vi "Main_05A.vi"() -> ()   [LabVIEW 2024]
panel:
  out "Page Array":cluster{"Array":i32[]}[](array[cluster])
  out "Rules":i32[][](array[numeric])
  out "Answer 6267":u32
  in  "Puzzle":string="57|32\n67|77\n67|23\n54|27\n54|35\n54|99\n27|63\n27|83\n27|14\n27|47\n83|96\n83|25\n83|45\n83|33\n83|82\n46|81\n46|67\n46|27\n46|72\n46|21\n46|73\n85|54\n85|99\n85|98\n85|28\n85|53\n85|27\n85|63\n76|69\n76|21\n76|54\n76|48\n76|92\n76|81\n76|62\n76|23\n51|75\n51|68\n51|25\n51|72\n51|62\n51|96\n51|21\n51|11\n51|27\n24|77\n24|63\n24|76\n24|72\n24|51\n24|14\n24|39\n24|18\n24|62\n24|67\n77|53\n77|57\n77|75\n77|36\n77|11\n77|23\n77|69\n77|96\n77|85\n77|52\n77|81\n45|23\n45|73\n45|54\n45|81\n45|36\n45|27\n45|65\n45|96\n45|76\n45|33\n45|52\n45|46\n11|61\n11|19\n11|39\n11|94\n11|98\n11|54\n11|56\n11|92\n11|24\n11|27\n11|43\n11|69\n11|28\n18|43\n18|76\n18|47\n18|72\n18|39\n18|25\n18|63\n18|14\n18|62\n18|32\n18|67\n18|94\n18|96\n18|77\n33|77\n33|36\n33|54\n33|73\n33|96\n33|75\n33|28\n33|23\n33|11\n33|81\n33|68\n33|65\n33|46\n33|52\n33|85\n36|69\n36|65\n36|52\n36|75\n36|48\n36|76\n36|54\n36|19\n36|68\n36|81\n36|57\n36|73\n36|56\n36|62\n36|21\n36|92\n52|73\n52|48\n52|85\n52|83\n52|23\n52|27\n52|57\n52|11\n52|31\n52|92\n52|28\n52|19\n52|54\n52|75\n52|99\n52|65\n52|24\n63|33\n63|65\n63|32\n63|35\n63|52\n63|51\n63|62\n63|45\n63|72\n63|82\n63|46\n63|96\n63|77\n63|47\n63|67\n63|23\n63|36\n63|14\n73|27\n73|99\n73|21\n73|63\n73|92\n73|98\n73|83\n73|85\n73|69\n73|39\n73|54\n73|11\n73|53\n73|32\n73|61\n73|19\n73|18\n73|57\n73|48\n19|24\n19|47\n19|82\n19|32\n19|46\n19|39\n19|92\n19|14\n19|33\n19|69\n19|83\n19|94\n19|48\n19|18\n19|57\n19|61\n19|51\n19|99\n19|56\n19|63\n99|72\n99|13\n99|14\n99|96\n99|82\n99|76\n99|35\n99|18\n99|61\n99|46\n99|39\n99|36\n99|33\n99|77\n99|51\n99|67\n99|47\n99|43\n99|94\n99|63\n99|24\n47|72\n47|52\n47|75\n47|65\n47|14\n47|96\n47|46\n47|11\n47|33\n47|85\n47|73\n47|67\n47|51\n47|82\n47|81\n47|13\n47|25\n47|77\n47|76\n47|36\n47|23\n47|62\n35|72\n35|65\n35|81\n35|47\n35|36\n35|52\n35|75\n35|62\n35|45\n35|96\n35|33\n35|46\n35|67\n35|13\n35|77\n35|76\n35|85\n35|23\n35|73\n35|51\n35|25\n35|14\n35|68\n94|13\n94|47\n94|68\n94|65\n94|82\n94|51\n94|36\n94|43\n94|67\n94|76\n94|46\n94|96\n94|35\n94|45\n94|81\n94|33\n94|72\n94|62\n94|14\n94|23\n94|25\n94|77\n94|52\n94|73\n69|82\n69|83\n69|61\n69|43\n69|35\n69|46\n69|63\n69|25\n69|67\n69|14\n69|47\n69|33\n69|24\n69|32\n69|56\n69|39\n69|72\n69|51\n69|94\n69|92\n69|48\n69|99\n69|45\n69|18\n96|62\n96|75\n96|73\n96|85\n96|57\n96|65\n96|69\n96|31\n96|23\n96|76\n96|19\n96|36\n96|81\n96|11\n96|53\n96|28\n96|27\n96|56\n96|68\n96|52\n96|21\n96|48\n96|98\n96|54\n61|13\n61|52\n61|62\n61|67\n61|35\n61|51\n61|82\n61|39\n61|36\n61|77\n61|45\n61|63\n61|32\n61|76\n61|14\n61|72\n61|94\n61|47\n61|46\n61|43\n61|33\n61|18\n61|96\n61|25\n68|21\n68|98\n68|18\n68|83\n68|57\n68|28\n68|73\n68|53\n68|99\n68|19\n68|69\n68|63\n68|11\n68|92\n68|85\n68|27\n68|48\n68|39\n68|61\n68|75\n68|56\n68|54\n68|24\n68|31\n53|82\n53|47\n53|69\n53|24\n53|32\n53|61\n53|63\n53|31\n53|39\n53|14\n53|92\n53|18\n53|98\n53|56\n53|83\n53|19\n53|99\n53|33\n53|94\n53|57\n53|35\n53|48\n53|45\n53|43\n23|24\n23|21\n23|28\n23|65\n23|73\n23|48\n23|98\n23|75\n23|31\n23|92\n23|19\n23|69\n23|56\n23|68\n23|53\n23|85\n23|57\n23|99\n23|27\n23|83\n23|81\n23|61\n23|11\n23|54\n21|98\n21|92\n21|31\n21|48\n21|43\n21|57\n21|35\n21|69\n21|56\n21|82\n21|39\n21|63\n21|94\n21|61\n21|53\n21|47\n21|28\n21|19\n21|24\n21|27\n21|83\n21|18\n21|99\n21|32\n72|11\n72|53\n72|76\n72|52\n72|85\n72|68\n72|13\n72|19\n72|27\n72|54\n72|23\n72|57\n72|36\n72|31\n72|21\n72|28\n72|73\n72|77\n72|98\n72|96\n72|81\n72|75\n72|65\n72|62\n14|72\n14|73\n14|77\n14|76\n14|52\n14|25\n14|11\n14|96\n14|51\n14|65\n14|67\n14|62\n14|13\n14|36\n14|21\n14|75\n14|68\n14|33\n14|81\n14|23\n14|46\n14|85\n14|45\n14|54\n98|43\n98|56\n98|47\n98|61\n98|24\n98|39\n98|69\n98|63\n98|32\n98|57\n98|51\n98|33\n98|83\n98|18\n98|35\n98|82\n98|48\n98|94\n98|99\n98|92\n98|19\n98|46\n98|45\n98|14\n82|96\n82|81\n82|23\n82|14\n82|13\n82|76\n82|73\n82|68\n82|77\n82|75\n82|33\n82|65\n82|11\n82|72\n82|36\n82|46\n82|67\n82|52\n82|51\n82|25\n82|54\n82|85\n82|45\n82|62\n13|68\n13|81\n13|73\n13|65\n13|54\n13|57\n13|52\n13|28\n13|62\n13|76\n13|23\n13|75\n13|36\n13|53\n13|21\n13|56\n13|69\n13|98\n13|31\n13|96\n13|27\n13|85\n13|11\n13|19\n65|98\n65|24\n65|81\n65|73\n65|31\n65|48\n65|28\n65|11\n65|53\n65|99\n65|27\n65|19\n65|18\n65|92\n65|85\n65|21\n65|61\n65|54\n65|83\n65|69\n65|56\n65|75\n65|68\n65|57\n39|25\n39|96\n39|47\n39|65\n39|35\n39|33\n39|72\n39|36\n39|52\n39|77\n39|94\n39|45\n39|23\n39|13\n39|46\n39|76\n39|14\n39|82\n39|62\n39|32\n39|51\n39|67\n39|43\n39|63\n62|85\n62|28\n62|99\n62|23\n62|53\n62|19\n62|31\n62|81\n62|57\n62|54\n62|21\n62|48\n62|65\n62|83\n62|98\n62|75\n62|11\n62|52\n62|69\n62|56\n62|92\n62|27\n62|68\n62|73\n81|75\n81|28\n81|57\n81|56\n81|53\n81|48\n81|85\n81|11\n81|21\n81|92\n81|99\n81|68\n81|27\n81|24\n81|98\n81|61\n81|39\n81|31\n81|54\n81|83\n81|73\n81|18\n81|19\n81|69\n56|25\n56|35\n56|82\n56|32\n56|94\n56|67\n56|99\n56|33\n56|48\n56|18\n56|24\n56|47\n56|46\n56|39\n56|83\n56|72\n56|45\n56|61\n56|63\n56|77\n56|51\n56|43\n56|14\n56|92\n43|62\n43|72\n43|73\n43|51\n43|96\n43|35\n43|45\n43|33\n43|52\n43|67\n43|65\n43|46\n43|23\n43|68\n43|76\n43|14\n43|13\n43|82\n43|47\n43|81\n43|85\n43|25\n43|36\n43|77\n48|63\n48|33\n48|14\n48|32\n48|61\n48|18\n48|83\n48|43\n48|24\n48|45\n48|72\n48|13\n48|92\n48|51\n48|67\n48|47\n48|35\n48|99\n48|82\n48|94\n48|25\n48|77\n48|39\n48|46\n28|98\n28|14\n28|53\n28|56\n28|45\n28|24\n28|47\n28|69\n28|99\n28|82\n28|61\n28|39\n28|43\n28|18\n28|63\n28|31\n28|35\n28|32\n28|83\n28|92\n28|48\n28|94\n28|57\n28|19\n25|77\n25|28\n25|19\n25|75\n25|27\n25|76\n25|21\n25|31\n25|98\n25|23\n25|72\n25|54\n25|96\n25|85\n25|52\n25|81\n25|53\n25|62\n25|13\n25|68\n25|36\n25|11\n25|65\n25|73\n75|28\n75|53\n75|83\n75|69\n75|11\n75|99\n75|24\n75|31\n75|56\n75|21\n75|98\n75|54\n75|19\n75|32\n75|94\n75|61\n75|43\n75|18\n75|39\n75|48\n75|63\n75|92\n75|27\n75|57\n92|47\n92|25\n92|35\n92|83\n92|77\n92|67\n92|72\n92|51\n92|46\n92|24\n92|99\n92|32\n92|13\n92|82\n92|18\n92|63\n92|61\n92|33\n92|96\n92|94\n92|39\n92|43\n92|45\n92|14\n31|24\n31|35\n31|63\n31|83\n31|39\n31|57\n31|45\n31|94\n31|32\n31|43\n31|48\n31|18\n31|82\n31|56\n31|14\n31|98\n31|99\n31|69\n31|33\n31|47\n31|46\n31|92\n31|19\n31|61\n32|76\n32|65\n32|25\n32|33\n32|67\n32|68\n32|13\n32|82\n32|96\n32|47\n32|23\n32|52\n32|14\n32|72\n32|51\n32|94\n32|77\n32|43\n32|81\n32|46\n32|35\n32|36\n32|62\n32|45\n57|92\n57|45\n57|14\n57|63\n57|18\n57|33\n57|82\n57|47\n57|83\n57|99\n57|94\n57|35\n57|56\n57|25\n57|43\n57|69\n57|46\n57|61\n57|39\n57|51\n57|48\n57|24\n57|67\n67|25\n67|53\n67|65\n67|98\n67|27\n67|62\n67|13\n67|31\n67|75\n67|52\n67|72\n67|36\n67|11\n67|54\n67|73\n67|21\n67|81\n67|28\n67|76\n67|96\n67|85\n67|68\n54|56\n54|31\n54|69\n54|57\n54|98\n54|94\n54|61\n54|24\n54|92\n54|47\n54|53\n54|43\n54|19\n54|28\n54|18\n54|83\n54|32\n54|63\n54|21\n54|39\n54|48\n27|19\n27|24\n27|94\n27|35\n27|18\n27|56\n27|31\n27|99\n27|43\n27|82\n27|57\n27|39\n27|32\n27|98\n27|53\n27|28\n27|92\n27|48\n27|69\n27|61\n83|18\n83|67\n83|61\n83|13\n83|14\n83|94\n83|36\n83|72\n83|24\n83|39\n83|77\n83|35\n83|99\n83|43\n83|32\n83|51\n83|46\n83|63\n83|47\n46|25\n46|52\n46|36\n46|68\n46|13\n46|76\n46|96\n46|77\n46|11\n46|51\n46|75\n46|85\n46|28\n46|54\n46|23\n46|65\n46|62\n46|53\n85|94\n85|11\n85|21\n85|57\n85|69\n85|56\n85|24\n85|18\n85|31\n85|39\n85|92\n85|32\n85|83\n85|19\n85|48\n85|61\n85|75\n76|98\n76|52\n76|53\n76|85\n76|57\n76|68\n76|56\n76|28\n76|83\n76|19\n76|11\n76|65\n76|75\n76|31\n76|73\n76|27\n51|54\n51|36\n51|77\n51|52\n51|28\n51|23\n51|67\n51|13\n51|31\n51|76\n51|85\n51|81\n51|65\n51|53\n51|73\n24|94\n24|33\n24|25\n24|96\n24|32\n24|43\n24|35\n24|61\n24|13\n24|45\n24|82\n24|36\n24|46\n24|47\n77|31\n77|21\n77|76\n77|65\n77|98\n77|27\n77|54\n77|73\n77|28\n77|13\n77|19\n77|62\n77|68\n45|13\n45|51\n45|77\n45|68\n45|62\n45|72\n45|11\n45|75\n45|85\n45|67\n45|25\n45|21\n11|63\n11|21\n11|83\n11|35\n11|32\n11|53\n11|48\n11|57\n11|31\n11|99\n11|18\n18|35\n18|23\n18|33\n18|82\n18|51\n18|45\n18|13\n18|36\n18|52\n18|46\n33|13\n33|51\n33|21\n33|25\n33|72\n33|62\n33|67\n33|76\n33|27\n36|53\n36|27\n36|23\n36|98\n36|28\n36|85\n36|11\n36|31\n52|69\n52|53\n52|98\n52|21\n52|68\n52|81\n52|56\n63|13\n63|81\n63|43\n63|94\n63|76\n63|25\n73|28\n73|24\n73|75\n73|56\n73|31\n19|43\n19|67\n19|45\n19|35\n99|25\n99|45\n99|32\n47|68\n47|45\n35|82\n\n46,51,67,25,72,77,13,96,36,76,52,23,65,81,68,73,85,75,11,54,21,27,28\n68,73,85,75,11,54,21,28,31,19,57,69,56,48,92,83,99,24,61,18,39\n83,99,24,61,63,32,94,35,47,82,14,45,33,46,51,67,25,72,77,13,96\n19,81,75,36,27,96,11\n75,11,54,21,28,31,98,19,56,92,83,99,24,18,63,32,94\n62,23,85,75,27,31,19,48,83\n23,65,81,68,73,85,11,54,27,31,98,19,57,48,92,83,24\n61,39,63,32,43,35,47,45,33,46,67,72,77,96,36\n27,28,53,31,98,19,57,69,56,48,92,83,99,24,61,18,39,63,32,94,35,47,82\n57,54,31,27,28,21,68,48,23,53,19\n18,39,63,32,94,43,35,47,82,14,33,46,51,67,25,72,77,13,96,36,76,62,52\n28,69,76,56,23,21,98,68,96,65,75,11,36,54,27,53,19,85,73,57,62\n14,46,96,73,75\n96,36,76,62,23,81,68,73,85,75,11,54,27,53,31,98,57,69,56\n98,57,56,48,92,83,99,24,18,39,94,43,82,14,45,33,46\n57,83,39,53,99,85,19,18,56\n68,85,27,28,56,83,61,18,39\n31,98,19,57,69,56,48,92,83,99,24,61,18,39,32,94,43,35,47,82,14,45,33\n62,39,13,43,72,36,82,45,61\n81,68,73,85,75,11,54,21,27,28,53,31,98,19,69,56,48,92,83,99,24,61,18\n61,18,45,56,83,47,43,63,35,39,69,92,25\n73,53,81,28,19,52,31,57,62,83,68,92,85,23,48\n52,23,65,81,68,73,85,75,11,54,21,27,28,53,31,98,19,69,56,48,92,83,99\n62,68,36,72,54,11,75,67,65\n24,39,63,32,47,14,45,33,46,67,25,77,96,36,76\n27,57,28,19,61,56,83,54,63,69,39,53,32,31,11\n43,14,46,51,72,77,36,65,81,68,73\n51,85,81,46,35,47,68,33,82,76,25,62,67,52,23\n69,24,83,92,53,99,21,56,18,31,11,43,63,57,94,98,61,39,28,19,48,32,54\n75,27,31,98,19,56,48,92,94\n47,45,33,51,72,77,36,76,62,52,65,81,68\n32,35,47,82,14,51,67,25,72,13,96,62,52,23,81\n19,31,54,81,76,56,52,65,21,28,73,36,75,68,96,11,53,27,23,69,98,57,62\n65,81,68,73,85,54,21,27,28,31,98,19,57,69,56,48,92,83,99,24,61\n83,99,61,94,82,14,33,46,51,67,25\n36,76,65,68,54,21,53,19,48\n23,65,81,11,83\n33,67,96,36,68,85,54,21,27\n54,18,24,39,21,98,63,27,92,83,31,61,48,75,57,28,69,85,73,19,11\n54,21,28,57,69,56,92,99,24,61,18,39,32,43,35\n39,63,32,94,35,47,46,51,67,72,77,13,96,76,62,52,23\n68,65,31,54,25,36,73,85,27,28,67\n13,67,68,81,96\n81,73,75,11,54,27,53,31,98,19,57,56,48,92,24,61,18\n92,54,24,32,28,19,53,39,35\n63,92,13,99,83,45,51\n85,11,54,21,28,53,31,98,56,24,61,18,32\n19,56,48,83,63,46,51\n75,11,21,27,28,53,31,19,57,92,83,99,24,61,18,39,63,32,94\n46,65,82,94,68,23,36,72,45,47,52,33,51,62,13\n56,48,92,83,99,24,61,39,63,32,94,43,35,47,82,14,33,46,51,67,72\n67,25,72,77,13,96,36,76,52,23,65,81,68,73,85,75,11,54,21,27,28,53,31\n83,57,31,54,21,92,28,85,63,53,48,39,73\n85,82,62,52,45,46,68,25,33\n25,27,21,68,98,72,81,23,13\n13,96,62,23,65,81,85,75,11\n98,57,11,73,99,52,48,65,28,75,19,85,69,92,83,81,56,21,31,68,27\n27,28,53,19,57,69,56,99,61,18,39,32,82\n53,21,48,54,28,68,36,73,85,76,23,31,98,11,81,56,52,57,69\n54,21,27,28,98,57,69,48,92,83,99,24,61,18,63,43,35\n23,65,81,68,27,57,24\n85,75,11,54,21,27,28,53,31,98,19,57,69,56,48,92,83,24,61,18,39,63,32\n54,53,27,11,56,39,68\n63,53,61,19,57,82,27\n14,76,51,43,46,82,67,45,52,35,96,94,33,81,47,13,65,36,77,62,23\n62,23,51,82,94,52,45,33,36,63,77,32,13,35,47,65,72,46,14,25,67,43,96\n92,83,99,24,61,18,39,32,94,43,35,47,82,14,45,33,46,51,67,25,72\n68,85,11,54,21,27,19,57,69,56,99,24,18\n48,18,83,46,82,77,67,72,24\n32,43,82,33,46,67,96,36,76\n28,65,11,68,54,27,23,56,98,92,19\n48,45,18,19,61,43,31,35,98,47,63,53,83,82,39,14,24,69,32,57,99\n92,83,99,24,18,39,32,94,35,82,51,72,13\n98,11,36,56,53,57,52,96,69,65,68\n33,77,96,76,62,52,23,65,68,75,54,21,27\n92,83,99,24,61,18,39,63,32,94,35,47,82,14,45,33,46,51,67,25,72,77,13\n33,67,13,96,62,65,73,85,27\n76,98,28,85,21\n75,28,31,98,57,92,99\n85,75,11,54,21,27,53,31,98,19,57,69,56,48,92,83,99,24,61,18,39,63,32\n72,76,62,65,81,75,11,21,53\n85,81,31,69,13,53,75,54,27,98,19,57,65\n94,35,47,82,14,45,33,46,51,67,25,72,77,13,96,36,76,62,52,23,65,81,68\n53,19,13,73,28,72,54,36,65,98,75\n76,11,62,68,53,77,65,54,28,75,52,85,21\n83,24,57,54,43,69,11\n23,82,35,52,43,39,13,77,47,63,96\n43,35,82,14,45,33,46,51,67,25,72,77,13,96,36,76,62,52,23,65,81,68,73\n36,19,13,98,65,76,23,81,28,72,11\n31,48,24,27,57,98,28,56,54,35,19\n21,13,85,31,27,57,36,68,81,54,76,96,73,77,23,52,62,11,75,19,98,65,53\n21,27,98,69,83,24,18,63,32,94,43,35,47\n56,99,69,48,54\n11,23,36,77,81,65,28,62,68,52,27,75,96,46,67\n83,24,61,18,63,94,43,35,47,82,14,46,51,67,25,77,96\n94,39,82,69,99,47,63,57,92,32,98,56,18,35,14,48,43,19,28\n72,76,96,67,65,73,82,68,35,52,85\n63,14,33,46,51,67,72\n63,32,94,43,35,82,14,46,51,72,77,96,36,76,62,23,65\n57,69,48,92,83,99,24,18,39,63,32,94,35,14,45,51,67\n57,99,61,39,47,82,46,51,67\n76,62,52,23,65,81,68,73,85,75,54,27,28,53,31,98,19,57,69,48,92\n75,36,21,85,46,28,27\n45,33,35,96,51,72,36,23,52,47,25,94,81,82,62,13,32,76,14\n11,54,21,28,53,98,19,57,69,56,92,83,99,24,61,39,32,94,43\n25,33,24,77,13,61,51,47,39,82,46,14,18,96,35,67,94,63,36,45,43,99,32\n85,13,68,53,27,36,69,57,52,11,96\n77,13,96,36,76,52,23,65,81,73,85,75,11,54,98,19,57\n47,67,72,13,62,52,68\n45,33,77,76,73\n39,92,18,35,72,13,61,82,77,32,51,14,46,47,45,25,63\n98,52,11,21,54,75,31,53,36,85,77,27,68,72,73,19,23,81,65\n45,25,82,11,68,52,85,75,23,46,51,96,77,67,72\n76,47,72,63,67,33,62,46,32,61,25,77,18,14,96,94,36,35,39,43,13\n76,62,52,65,81,21,28\n69,56,48,92,83,99,24,61,39,32,94,43,35,47,82,45,33,46,51,67,25\n85,81,23,77,54,72,51,76,36,75,21,68,11,67,28,13,65\n73,21,68,45,11,85,23,33,81,36,46\n67,24,45,83,32,39,61\n28,51,67,46,76,96,11,21,73,27,62,25,65,85,52\n13,36,52,23,81,54,31,57,69\n21,27,28,53,98,19,69,56,48,92,24,18,94,35,47\n24,18,39,63,32,94,35,47,82,14,45,33,46,67,25,72,77,13,96,36,76\n51,36,76,62,11,27,53\n81,68,73,54,21,28,53,98,57,69,48,92,83,99,24,61,18\n46,33,98,19,69,61,14,45,47,24,48,82,99,57,63,94,39,83,56\n28,57,92,83,24,39,63,35,14\n65,73,85,75,11,54,28,24,61\n48,92,83,99,24,61,47,72,77\n82,25,83,61,77,39,63,45,99\n36,76,65,73,54,56,48\n19,83,24,18,39,63,32,94,43,35,82,14,33,46,51\n11,21,53,69,56,48,83,32,43\n32,45,25,94,99,63,47,48,82,77,14\n32,57,46,33,24,14,69,83,82,51,39,92,99,63,61,48,67,47,18\n48,57,11,92,65,53,61,75,21,56,83,73,54,68,27,69,31,24,98,28,19,81,99\n31,75,83,62,57,68,52,23,56,73,48\n45,92,94,61,32,13,18\n46,27,76,52,62,68,36,33,54,21,72,96,51\n19,57,69,56,48,92,99,24,61,18,39,63,32,94,43,35,47,82,14,45,33,46,51\n69,83,99,24,61,39,63,94,35,82,45,33,51,67,25\n53,31,69,63,83,54,85,21,18,28,92,27,57,98,48,24,56,75,32,39,99,61,19\n81,82,35,72,96,68,36,46,13,62,14,73,76,25,33,52,43,67,45\n69,56,48,61,35,82,14,45,25\n76,23,81,11,21,28,19,57,48\n73,75,11,21,27,53,98,19,57,69,56,83,99,24,61,18,39\n18,39,63,32,94,43,35,47,82,14,45,46,51,67,25,72,77,13,36,62,52\n94,69,99,56,43,46,61,63,67,82,35,47,32,83,18,39,48,92,51,24,45,33,25\n27,56,81,11,53,18,68,69,48\n61,35,13,94,77,47,51,99,63,18,36,67,24,45,46,43,72,32,33,96,14,39,25\n32,57,28,53,99,27,18,75,48,85,83\n32,43,47,14,51,67,25,13,36,76,52\n73,75,54,21,53,98,19,48,83,99,61\n76,52,81,68,28\n75,98,56,83,39\n43,33,36,67,62,72,18,94,77,45,35,82,32,61,76,96,14\n54,21,27,53,98,69,56,92,83,99,18,39,63,32,94,43,35\n53,75,56,21,99,85,83,19,92,73,48,28,31,23,11,57,81\n21,28,53,98,69,24,63\n48,99,43,94,92,53,82,69,27,56,39,32,35\n24,18,39,94,43,35,47,82,14,45,33,46,51,67,25,13,96,36,76\n65,14,25,77,54,33,23,52,96,13,11,68,73\n92,57,94,53,19,63,98,47,99,18,61,39,82,14,24,35,69,28,83,56,32,48,43\n94,39,48,83,99,53,69,31,14,28,98,82,32,18,24,35,63,56,47,61,92,19,57\n25,72,77,13,96,36,76,62,52,23,65,81,68,73,85,75,11,54,27,28,53,31,98\n36,76,62,52,23,65,81,73,75,11,54,53,98,19,57\n56,48,35,43,45,18,72,63,83\n68,62,31,67,73,72,23,13,81,76,36\n21,28,98,57,39,54,19,61,18,92,83,24,11,63,69,43,94\n25,13,96,76,62,52,81,73,85,75,11,54,27,31,98\n62,65,81,68,73,75,54,27,28,57,69,92,83\n45,47,62,35,46,32,82,14,96,52,39,67,94,33,25,77,36,72,13,51,43,18,63\n36,82,67,96,35,62,94,43,61,13,46,51,47,77,18,76,39,25,63,14,33,45,32\n19,57,69,56,48,83,99,24,61,18,39,63,94,43,47,82,14,45,33,46,51\n28,81,75,11,72,98,62,68,65,52,19\n82,33,65,76,51,45,72,36,96,77,63,32,13,94,47\n48,83,99,63,43,35,77\n21,27,28,53,31,19,57,69,56,48,92,83,99,24,61,18,39,63,32,94,43,35,47\n35,25,36,47,18,24,14,77,99,45,96\n96,11,23,13,85,76,73,33,65,21,67,52,36,81,25,27,62\n82,45,33,67,62,65,73\n14,36,61,94,43\n76,27,92,28,75,52,69\n31,56,28,68,73,69,57,53,21,23,11,65,76,62,48,75,54,19,98,92,27,52,85\n36,76,52,23,65,81,68,73,85,75,11,54,21,27,28,53,31,98,19,57,69,56,48\n99,61,18,43,53,45,47,83,24,94,63,92,56,57,82,69,14\n82,94,57,14,83,32,46,35,98,99,45\n53,98,19,57,69,56,48,92,24,39,63,32,94,43,35,47,82,14,45\n35,82,14,45,33,46,25,72,77,96,23,65,85\n98,92,81,53,85,76,48,27,62\n98,57,92,99,18,39,43,47,82,14,45,33,46\n28,53,31,98,57,69,48,83,99,24,61,18,39,63,32,43,35,47,82\n24,61,39,63,32,35,46,51,67,36,76\n99,98,33,18,82,48,24,45,35,32,19\n62,52,23,81,68,73,85,75,11,54,21,53,98,19,57,56,48,92,83\n73,28,53,19,56,99,24\n81,45,82,14,43,73,46,47,33,68,77,96,25,51,13,35,23,52,62\n65,28,61,83,99,92,98\n83,99,94,43,47,67,96\n82,14,46,51,67,77,96,76,23,85,75\n45,46,51,81,75\n94,43,35,47,82,14,45,46,67,72,13,96,36,52,65\n81,77,11,28,31,68,85,54,76,65,62,36,75,21,57,19,98,27,52,23,96\n83,54,21,18,39,68,53\n33,18,69,51,24,94,14,19,48\n32,36,94,13,67,51,35,46,62,96,63,77,72,52,76,82,23\n76,62,52,23,65,81,68,73,85,11,27,28,98,57,48\n69,56,48,92,24,18,39,94,43,35,82,45,33,67,25\n46,51,67,25,72,77,13,96,76,62,52,23,68,73,85,75,11,54,21,27,28"
  in  "Example":string="47|53\n97|13\n97|61\n97|47\n75|29\n61|13\n75|53\n29|13\n97|29\n53|29\n61|53\n97|53\n61|29\n47|13\n75|47\n97|75\n47|61\n75|61\n47|29\n75|13\n53|13\n\n75,47,61,53,29\n97,61,53,29,13\n75,29,13\n75,97,47,61,53\n61,13,29\n97,13,75,29,47"
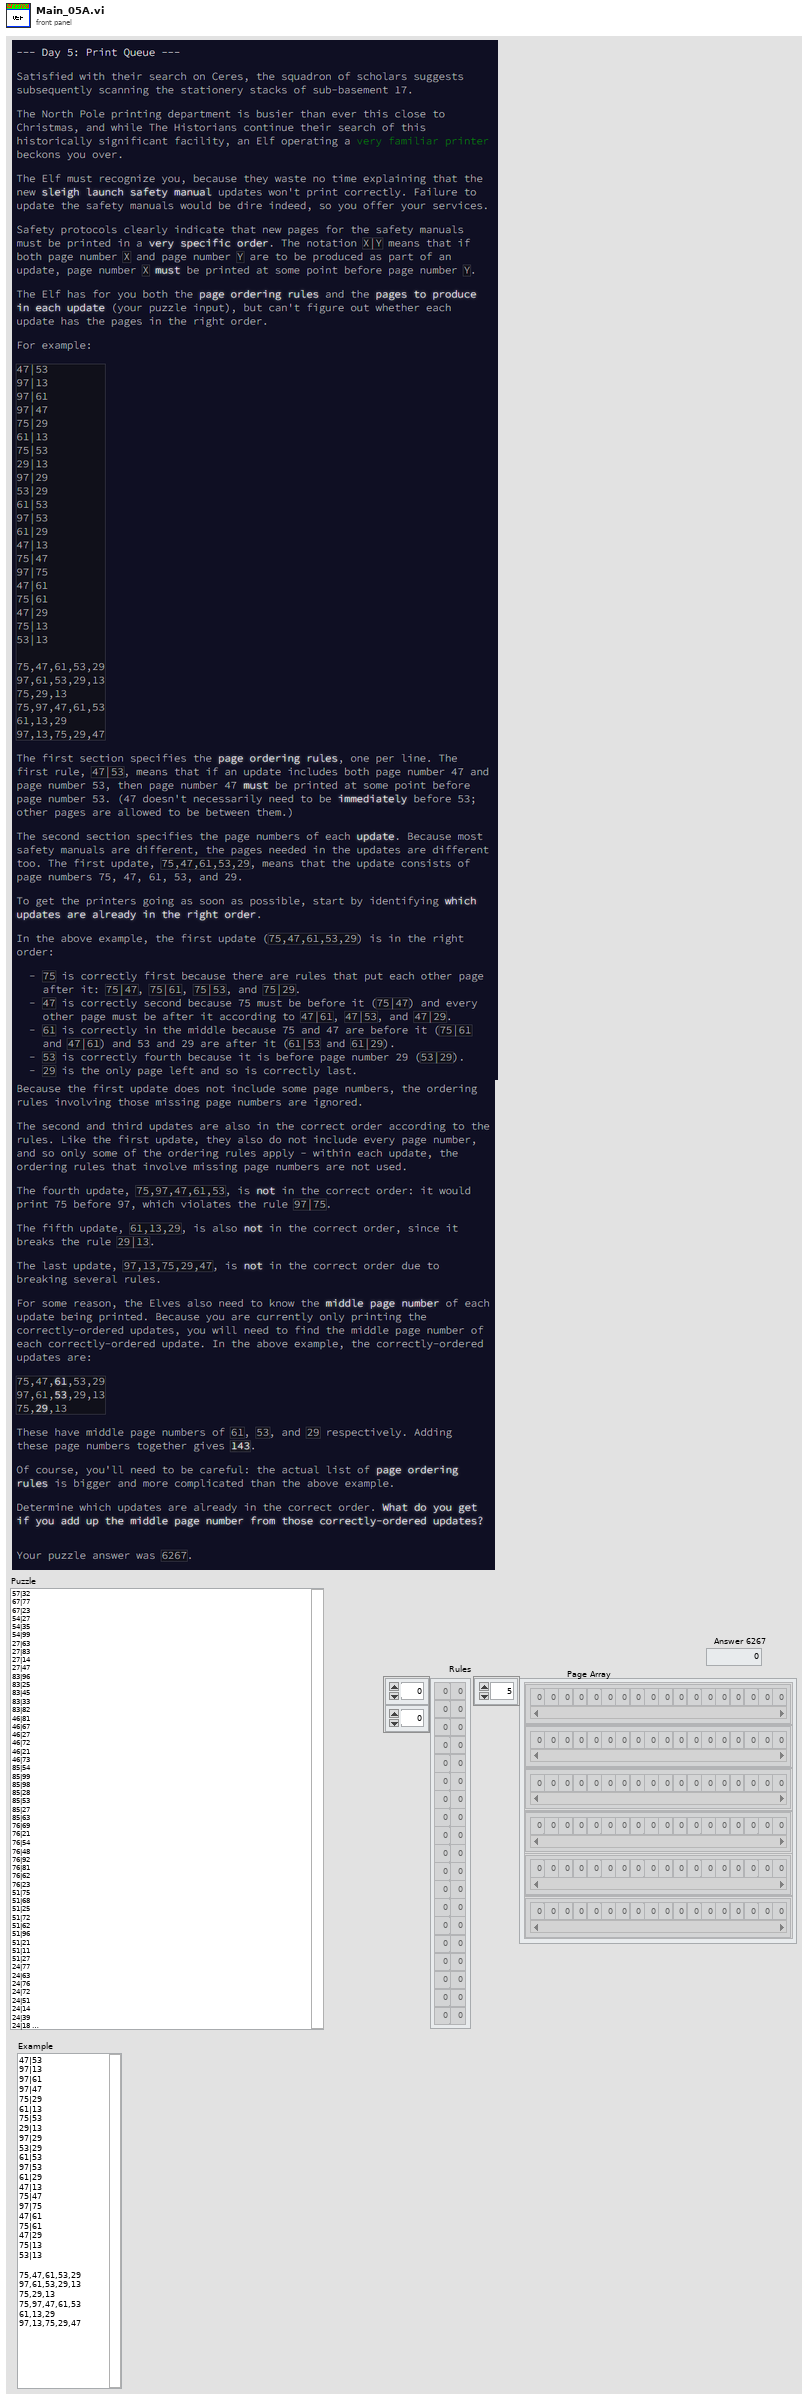
[diagram p1: front panel]
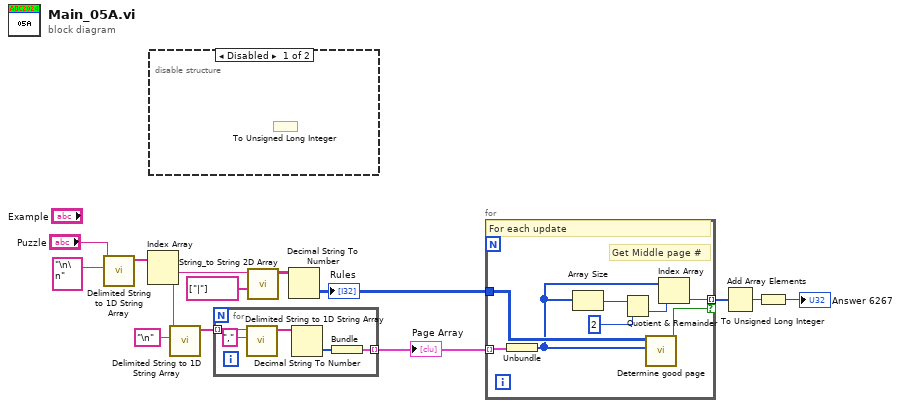
[diagram p0: block diagram]
diagram:
  n1 = call <vilib>:"Delimited String to 1D String Array.vi"("delimiter"="\n\n" ("delimiter (Tab)"), "delimited string"="Puzzle") -> ("string array"=w13:string[])  [unwired: 9 in]
  n2 = Index Array(array=w13) -> (element #1=w12:string, element #2=w9:string)  [unwired: 2 in]
  n3 = disable-structure shown="Disabled" {
    frame Disabled {
      n4 = To Unsigned Long Integer() -> ()  [unwired: 1 in, 1 out]
    }
    frame Enabled {
    }
  }
  n5 = call <vilib>:"Delimited String to 1D String Array.vi"("delimiter"="\n", "delimited string"=w9) -> ("string array"=w7:string[])  [unwired: 9 in]
  n6 = for {
    tunnel: w7 -> [w19] mode=indexing
    tunnel: [w15] -> w6 mode=indexing
    n7 = call <vilib>:"Delimited String to 1D String Array.vi"("delimiter"=",", "delimited string"=w19) -> ("string array"=w17:string[])  [unwired: 9 in]
    n8 = Decimal String To Number(string=w17) -> (number=w16:i32[])  [unwired: 2 in, 1 out]
    n9 = Bundle(w16) -> (w15:cluster{i32[]})  [unwired: 1 in]
  }
  "Page Array" <- w6
  n10 = call "String_to String 2D Array.vi"("Seperators Column ()"=string[] ["|"], "Input String"=w12) -> ("2D Array"=w10:string[][])  [unwired: 9 in]
  n11 = Decimal String To Number(string=w10) -> (number=w5:i32[][])  [unwired: 2 in, 1 out]
  "Rules" <- w5
  n12 = for {
    tunnel: w6 -> [w27] mode=indexing
    tunnel: w5 -> [w26]
    tunnel: [w21] -> w2 mode=indexing if=w20
    # "Get Middle page #"
    # "For each update"
    n13 = Unbundle(w27) -> (w23:i32[])
    n14 = Array Size(array=w23) -> (size(s)=w25:i32)
    n15 = Quotient & Remainder(x=w25, y=2) -> (floor(x/y)=w22:i32)  [unwired: 1 out]
    n16 = call "Determine good page.vi"("Page"=w23, "Rules"=w26) -> ("Correct Order Out"=w20:bool)  [unwired: 9 in]
    n17 = Index Array(array=w23, index=w22) -> (element=w21:i32)
  }
  n18 = Add Array Elements(numeric array=w2) -> (sum=w4:i32)
  n19 = To Unsigned Long Integer(number=w4) -> (unsigned 32bit integer=→"Answer 6267":u32)
